vi "Perform_Meas_Setup.vi"(2 "Simulate/Run":T1, 3 "Traverse line":T2 {"Row Duration (mins)" format="%#.1f"; "Row No" min=0; "Trace Gas Concentration (%)" min=0.0 format="%#.2f"; "Emission Rate (l/min)" format="%#.2f"; "Tunnel Speed" format="%#.2f"; "Start X" format="%#.2f"; "Start Y" format="%#.2f"; "Start Z" format="%#.2f"; "End X" format="%#.2f"; "End Y" format="%#.2f"; "End Z" format="%#.2f"; "Averaging time (min)" min=0.0 format="%#.1f"}) -> (0 "Continue?":bool)   [LabVIEW 2010]
uses:
  Traverse_cluster.ctl
  Spacing.ctl
  Controls/Multi_run_mode.ctl
  Controls/User_Specific_mode.ctl
  Controls/Save_Data.ctl
  Controls/Setup.ctl
  Globals/Constants_global.vi
panel:
  # "X           Y            Z"
  # "Start"
  # "End"
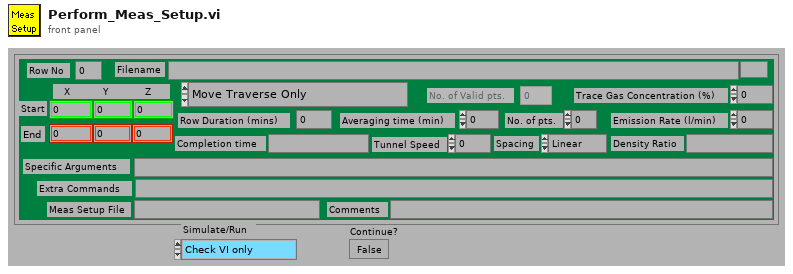
[diagram p1: front panel]
types:
  T1 = typedef "User_Specific_mode.ctl" = enum16{"Check VI only", "Run VI"}
  T2 = typedef "Traverse_cluster.ctl" = cluster{"Start X":dbl, "Start Y":dbl, "Start Z":dbl, "End X":dbl, "End Y":dbl, "End Z":dbl, "No. of pts.":i32, "Spacing":T3, "Filename":path, "Tunnel Speed":dbl, "Averaging time (min)":dbl, "Extra Commands":string, "Specific Arguments":string, "Emission Rate (l/min)":dbl, "Trace Gas Concentration (%)":dbl, "Density Ratio":string, "Comments":string, "Row No":i32, "Row Type Selector":T4, "Completion time":string, "Row Duration (mins)":dbl, "No. of Valid pts.":i32, "Meas Setup File":string}
  T3 = typedef "Spacing.ctl" = enum16{"Linear", "Log", "Gauss", "Specified", "N/A"}
  T4 = typedef "Multi_run_mode.ctl" = enum16{"Move Traverse Only", "Set Tunnel Speed Only", "Set Source Only", "Set Measurement Conditions", "Single Measurement", "Vertical Profile", "Lateral Profile", "Longitudinal Profile", "Explore Volume", "Multi-Axis Profile", "Auto Calibrate", "Meas Fast FID Bkgnd", "Check Beam Power", "Scanning Valve Measurement", "Run VI Named:", "Set ADAM Ch", "Wait (minutes)", "Send Message", "Synchronize With:", "Fall Back to this Row", "Turn Off Row Repeating", "Blank Row"}
  T5 = typedef "Save_Data.ctl" = enum16{"Save No Data", "Save Data"}
  T6 = typedef "Setup.ctl" = enum16{"Run Program", "Show Setup", "Save Current Setup", "Setup Front Panel"}
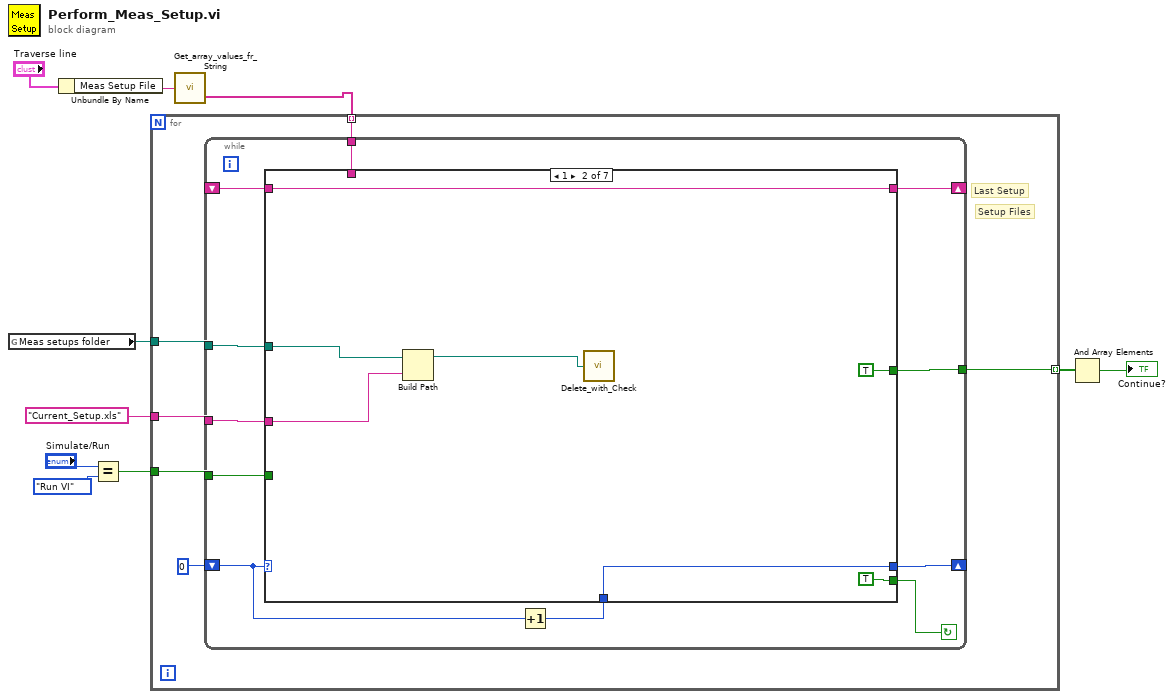
[diagram p0: block diagram]
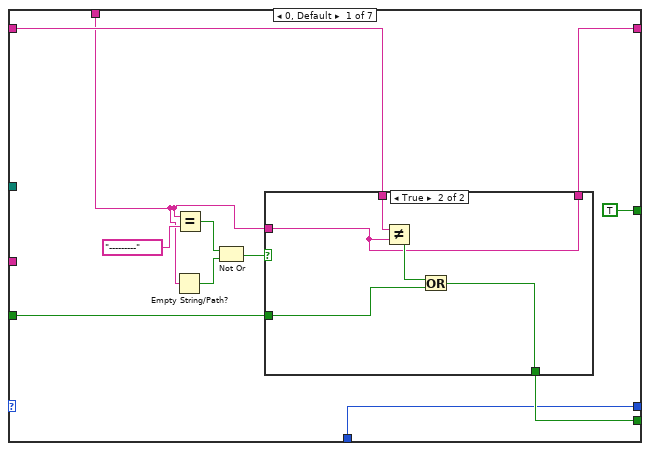
[diagram p2: hidden frame]
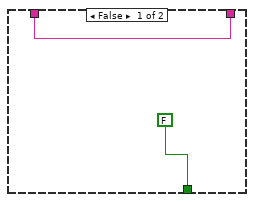
[diagram p3: hidden frame]
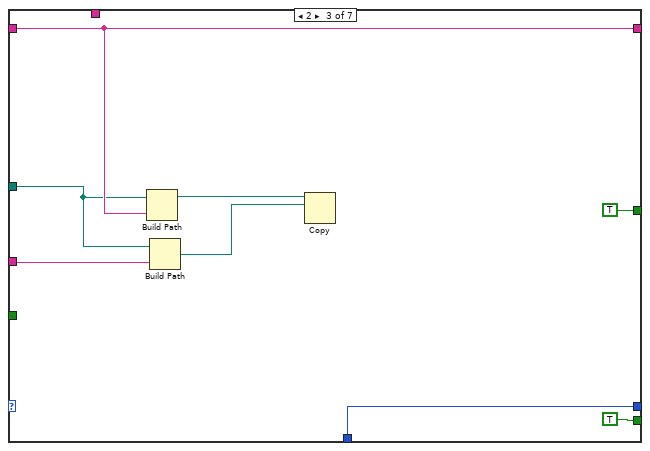
[diagram p4: hidden frame]
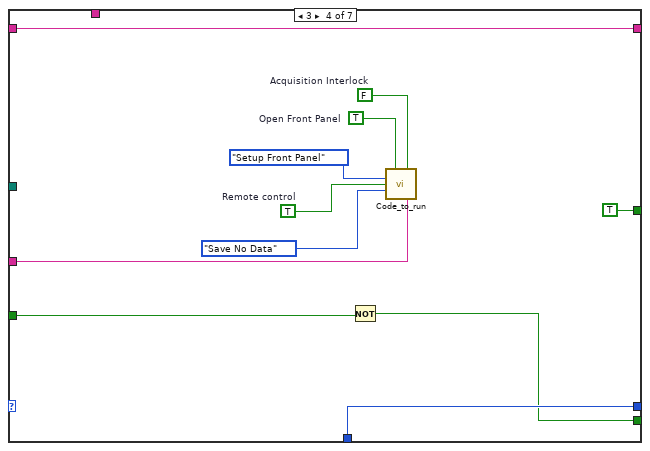
[diagram p5: hidden frame]
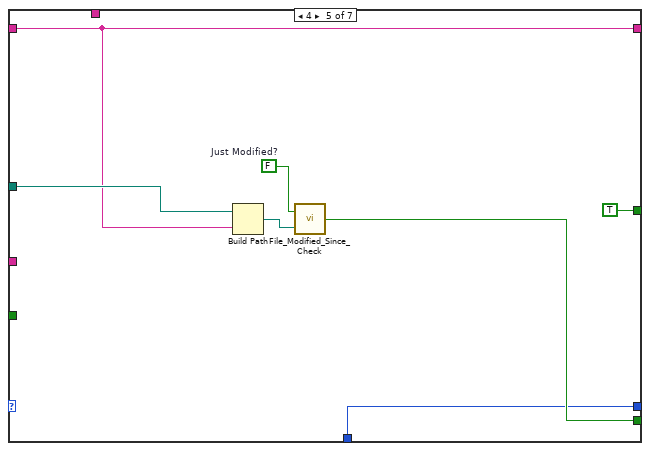
[diagram p6: hidden frame]
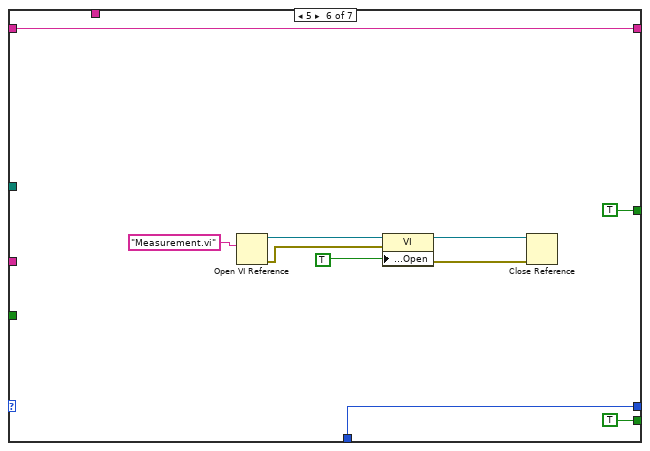
[diagram p7: hidden frame]
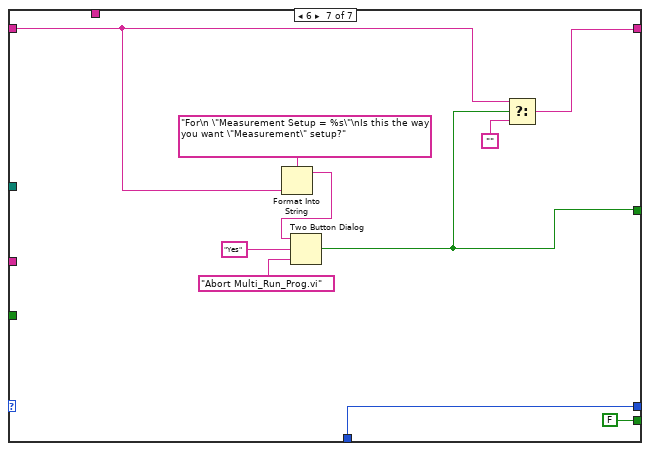
[diagram p8: hidden frame]
diagram:
  n1 = global read "Constants_global.vi" "Meas setups folder"() -> (w10:path)
  n2 = Unbundle By Name("Traverse line") -> ("Meas Setup File"=w4:string)
  n3 = Equal?(x="Simulate/Run", y=User_Specific_mode."Run VI" ("Simulate/Run")) -> (x = y?=w6:bool)
  n4 = call "Get_array_values_fr_String.vi"("String Value"=w4) -> ("String array"=w3:string[])  [unwired: 1 out]
  n5 = for {
    tunnel: w10 -> [w16]
    tunnel: "Current_Setup.xls" ("name or relative path") -> [w14]
    tunnel: w6 -> [w13]
    tunnel: w3 -> [w12] mode=indexing
    tunnel: [w11] -> w2 mode=indexing
    # "Last Setup"
    # "Setup Files"
    n6 = while {
      tunnel: w13 -> [w18]
      tunnel: w14 -> [w19]
      tunnel: w16 -> [w20]
      shift-left: _ -> [w22]
      shift-right: [w21] -> _
      tunnel: [w23] -> w11
      shift-left: 0 -> [w26]
      shift-right: [w24] -> _
      tunnel: w12 -> [w17]
      stop <- w27 continue-if-true
      n7 = Increment(x=w26) -> (x+1=w25:i32)
      n8 = case shown="1" w26 {
        tunnel: [w35 TRUE ("T button?") TRUE ("T button?") w63 w76 TRUE FALSE] -> w27
        tunnel: w25 -> [w33 w49 w58 w65 w75 w88 w98]
        tunnel: [w33 w49 w58 w65 w75 w88 w98] -> w24
        tunnel: [TRUE ("T button?") TRUE ("T button?") TRUE ("T button?") TRUE ("T button?") TRUE ("T button?") TRUE ("T button?") w92] -> w23
        tunnel: w22 -> [w37 w51 w57 w67 w73 w87 w90]
        tunnel: [w36 w51 w57 w67 w73 w87 w91] -> w21
        tunnel: w20 -> [_ w48 w54 _ w77 _ _]
        tunnel: w19 -> [_ w47 w53 w66 _ _ _]
        tunnel: w18 -> [w34 _ _ w64 _ _ _]
        tunnel: w17 -> [w28 _ _ _ _ _ _]
        frame 0, Default {
          n9 = Empty String/Path?(string/path=w28) -> (empty?=w30:bool)
          n10 = Equal?(x=w28, y="---------" ("f")) -> (x = y?=w31:bool)
          n11 = Not Or(1:w30, 2:w31) -> (0:w29:bool)
          n12 = case shown="True" w29 {
            tunnel: [w40 w42] -> w36
            tunnel: w28 -> [_ w42]
            tunnel: w37 -> [w40 w45]
            tunnel: [FALSE w43] -> w35
            tunnel: w34 -> [_ w41]
            frame False {
            }
            frame True {
              n13 = Not Equal?(x=w45, y=w42) -> (x != y?=w44:bool)
              n14 = Or(x=w44, y=w41) -> (x .or. y?=w43:bool)
            }
          }
        }
        frame 1 {
          n15 = Build Path(base path=w48, name or relative path=w47) -> (appended path=w46:path)
          n16 = call "Delete_with_Check.vi"("FilePath"=w46) -> ()  [unwired: 1 out]
        }
        frame 2 {
          n17 = Build Path(base path=w54, name or relative path=w57) -> (appended path=w56:path)
          n18 = Build Path(base path=w54, name or relative path=w53) -> (appended path=w55:path)
          n19 = Copy(10:w55, 11:w56) -> ()  [unwired: 1 in, 5 out]
        }
        frame 3 {
          w68 = FALSE  # Acquisition Interlock
          w70 = TRUE  # Remote control
          w71 = TRUE  # Open Front Panel
          n20 = Not(x=w64) -> (.not. x?=w63:bool)
          n21 = call "Code_to_run.vi"("Open Front Panel"=w71, "Acquisition Interlock"=w68, "setup"=Setup."Setup Front Panel", "Remote control"=w70, "File"=Save_Data."Save No Data", "Setup filename"=w66) -> ()  [unwired: 4 in, 6 out]
        }
        frame 4 {
          w72 = FALSE  # Just Modified?
          n22 = Build Path(base path=w77, name or relative path=w73) -> (appended path=w78:path)
          n23 = call "File_Modified_Since_Check.vi"("Pathname"=w78, "Just Modified?"=w72) -> ("Modified?"=w76:bool)
        }
        frame 5 {
          n24 = Open VI Reference(vi path="Measurement.vi") -> (vi reference=w83:refnum<vi>, error out=w84:errorcluster)  [unwired: 1 in, 4 out]
          n25 = property class="VI"(reference=w83, error in=w84, "Front Panel Window:Open"=TRUE) -> (reference out=w81:refnum<vi>, error out=w80:errorcluster)
          n26 = Close Reference(reference=w81, error in (no error)=w80) -> ()  [unwired: 1 out]
        }
        frame 6 {
          n27 = Format Into String(format string="For\n \"Measurement Setup = %s\"\nIs this the way you want \"Measurement\" setup?" ("message"), w90) -> (resulting string=w97:string)  [unwired: 2 in, 1 out]
          n28 = Two Button Dialog(message=w97, 1:"Abort Multi_Run_Prog.vi" ("F button name (\"Cancel\")"), 2:"Yes" ("T button name (\"OK\")")) -> (T button?=w92:bool)
          n29 = Select(t=w90, s=w92, f="") -> (s? t:f=w91:string)
        }
      }
    }
  }
  n30 = And Array Elements(Boolean array=w2) -> (logical AND=→"Continue?":bool)
